vi "GetImageHeads.vi"(10 "Offsets":i32[](array[numeric]), 11 "RefIn":refnum<file>) -> (0 "HeightHead":T1, 1 "IntensityHead":T1, 2 "LaserOpticalHead":T1, 3 "OpticalHead":T1, 4 "RefOut":refnum<file>)   [LabVIEW 2014]
uses:
  ImageHeaderType.ctl
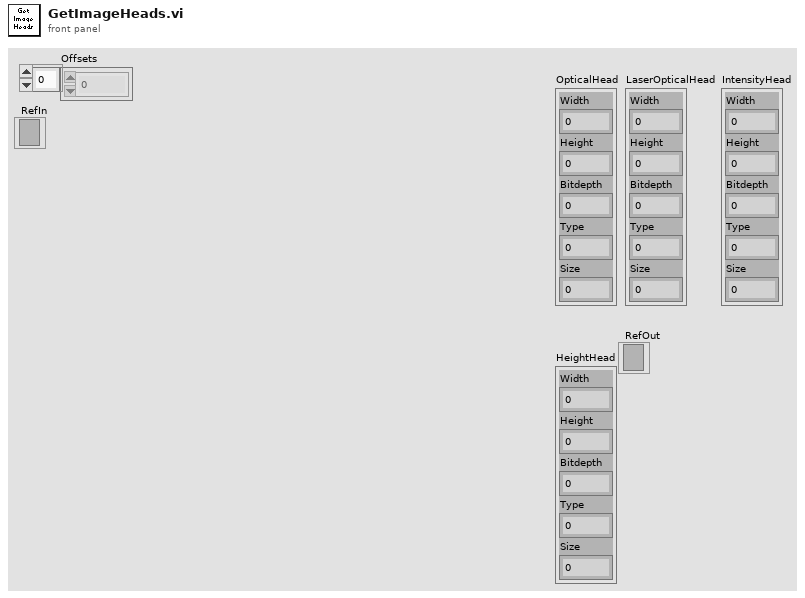
[diagram p1: front panel]
types:
  T1 = typedef "ImageHeaderType.ctl" = cluster{"Width":u32, "Height":u32, "Bitdepth":u32, "Type":u32, "Size":u32}
  T2 = enum16{"big-endian, network order", "native, host order", "little-endian"}
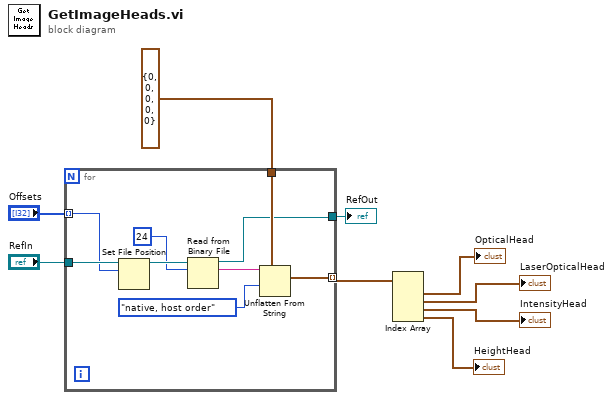
[diagram p0: block diagram]
diagram:
  n1 = for {
    tunnel: "RefIn" -> [w18]
    tunnel: "Offsets" -> [w15] mode=indexing
    tunnel: [w13] -> w9 mode=indexing
    tunnel: T1 {"Width"=0, "Height"=0, "Bitdepth"=0, "Type"=0, "Size"=0} ("ImageHeader") -> [w11]
    tunnel: [w10] -> w1
    n2 = Set File Position(offset (in bytes) (0)=w15, refnum=w18) -> (refnum out=w17:refnum<file>)  [unwired: 2 in, 1 out]
    n3 = Read from Binary File(10:24 ("count (1)"), 11:w17) -> (2:w14:string, 3:w10:refnum<file>)  [unwired: 4 in, 2 out]
    n4 = Unflatten From String(type=w11, binary string=w14, byte order (0:big-endian, network order)=T2."native, host order") -> (value=w13:T1)  [unwired: 2 in, 2 out]
  }
  "RefOut" <- w1
  n5 = Index Array(array=w9) -> (element #1=→"OpticalHead":T1, element #2=→"LaserOpticalHead":T1, element #3=→"IntensityHead":T1, element #4=→"HeightHead":T1)  [unwired: 4 in]
